vi "Insert.vi"(8 "error in (no error)":errorcluster, 9 "Item":refnum<class>, 10 "Index":i32, 11 "BufferedArray in":refnum<class "BufferedArray.lvclass">) -> (0 "error out":errorcluster, 3 "BufferedArray out":refnum<class "BufferedArray.lvclass">)   [LabVIEW 2013, in "LapDog.Collections.v_.Lists.Implementations.lvlib" / "BufferedArray.lvclass"]
doc: "Inserts an item into the list at the location specified by Index, increasing the index of all items after the specified index by 1. If Index = -1 or Index = Count, the item is added to the end of the list. If Index < -1 or Index > Count, error 510201 is returned."
uses:
  BufferedArray.lvclass
  LapDog.Collections.Common/LapDog.Collections.v_.Common.lvlib
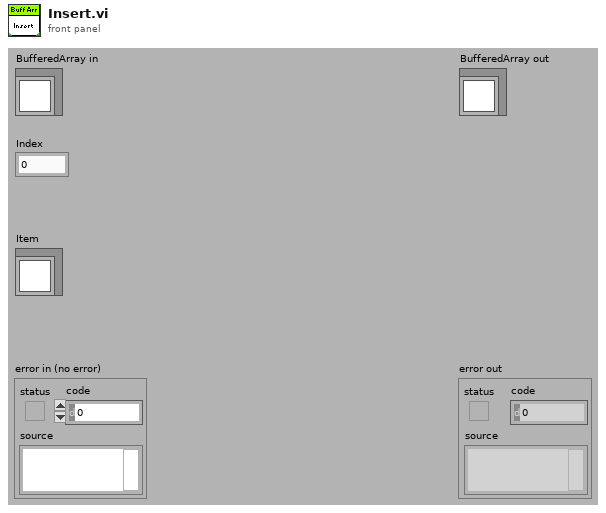
[diagram p1: front panel]
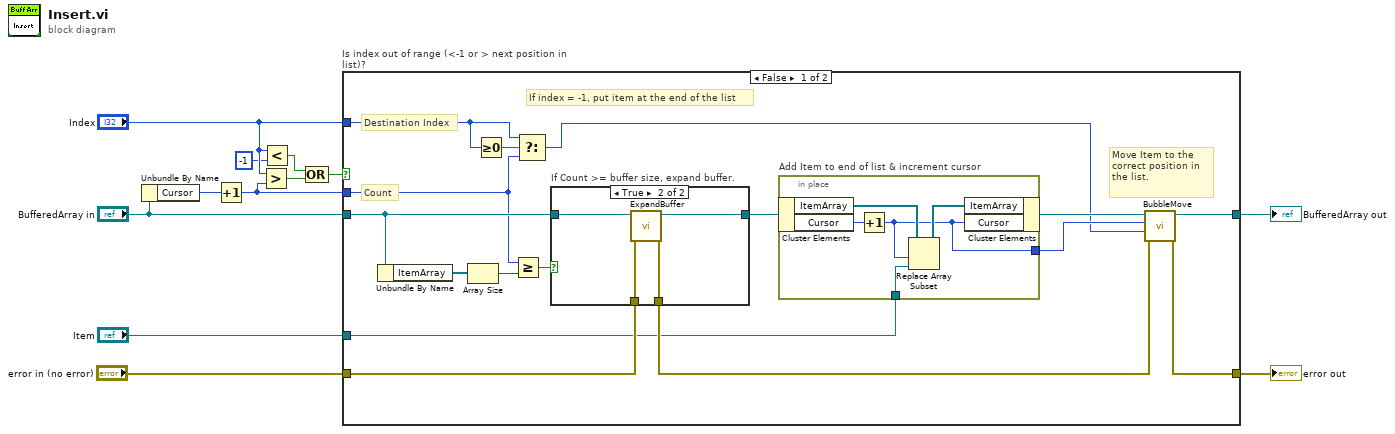
[diagram p0: block diagram]
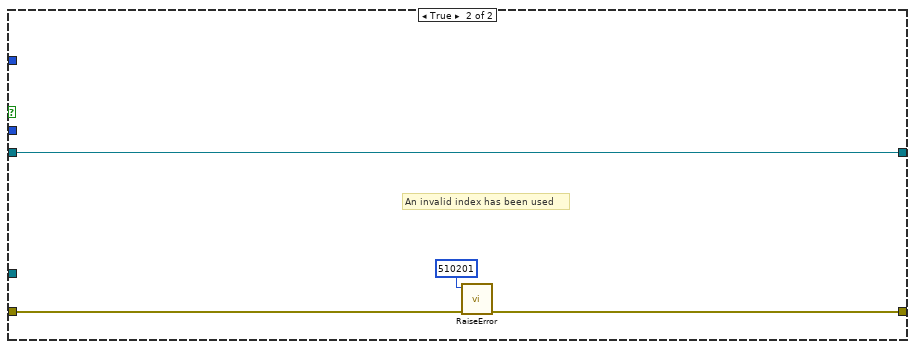
[diagram p3: hidden frame]
diagram:
  n1 = Unbundle By Name("BufferedArray in") -> ("Cursor"=w7:i32)
  n2 = Increment(x=w7) -> (x+1=w8:i32)
  n3 = Greater?(x="Index", y=w8) -> (0:w2:bool)
  n4 = Less?(x="Index", y=-1) -> (x < y?=w3:bool)
  n5 = Compound Arithmetic op=OR(w3, w2) -> (w1:bool)
  n6 = case "Is index out of range (<-1 or > next position in list)?" shown="False" w1 {
    tunnel: [w23 w43] -> w12
    tunnel: "error in (no error)" -> [w25 w41]
    tunnel: [w21 w40] -> w10
    tunnel: "BufferedArray in" -> [w24 w43]
    tunnel: w8 -> [w15 _]
    tunnel: "Index" -> [w14 _]
    tunnel: "Item" -> [w18 _]
    frame False {
      # "If index = -1, put item at the end of the list"
      # "Move Item to the correct position in the list."
      # "Destination Index"
      # "Count"
      n7 = Unbundle By Name(w24) -> ("ItemArray"=w28:refnum<class>[])
      n8 = Array Size(array=w28) -> (size(s)=w27:i32)
      n9 = Greater Or Equal To 0?(x=w14) -> (x >= 0?=w16:bool)
      n10 = Greater Or Equal?(x=w15, y=w27) -> (x >= y?=w26:bool)
      n11 = Select(t=w14, s=w16, f=w15) -> (s? t:f=w13:i32)
      n12 = case "If Count >= buffer size, expand buffer." shown="True" w26 {
        tunnel: w24 -> [w35 w39]
        tunnel: [w35 w38] -> w20
        tunnel: w25 -> [w34 w37]
        tunnel: [w34 w36] -> w22
        frame False {
        }
        frame True {
          n13 = call-dynamic "ExpandBuffer.vi"("error in (no error)"=w37, "BufferedArray in"=w39) -> ("error out"=w36:errorcluster, "BufferedArray out"=w38:refnum<class "BufferedArray.lvclass">)  [unwired: 8 in]
        }
      }
      n14 = in-place "Add Item to end of list & increment cursor" {
        in-place-border: w18 -> [w30]
        in-place-border: [w29] -> w17
        n15 = in-place-cluster #1(w20) -> ("ItemArray"=w33:refnum<class>[], "Cursor"=w31:i32)
        n16 = Increment(x=w31) -> (x+1=w29:i32)
        n17 = Replace Array Subset(array=w33, new element=w30, index=w29) -> (w32:refnum<class>[])
        n18 = in-place-cluster #1("ItemArray"=w32, "Cursor"=w29) -> (w19:refnum<class "BufferedArray.lvclass">)
      }
      n19 = call "BubbleMove.vi"("error in (no error)"=w22, "Destination Index"=w13, "Current Index"=w17, "BufferedArray in"=w19) -> ("error out"=w21:errorcluster, "BufferedArray out"=w23:refnum<class "BufferedArray.lvclass">)  [unwired: 6 in]
    }
    frame True {
      # "An invalid index has been used"
      n20 = call "RaiseError.vi"("error in (no error)"=w41, "Error Code"=510201) -> ("error out"=w40:errorcluster)  [unwired: 9 in]
    }
  }
  "error out" <- w10
  "BufferedArray out" <- w12
